vi "Set User Object Tag.vi"(8 "error in (no error)":errorcluster, 9 "Value":variant, 10 "Tag Name":string, 11 "Generic Refnum":refnum<vi>) -> (0 "error out":errorcluster, 1 "Was Tag Set?":bool, 3 "dup Generic Refnum":refnum<vi>)   [LabVIEW 2020, in "UserTags.lvlib"]
doc: "UserTags.lvlib contains VIs that allow you to store data within objects or VIs as \"tags\". You can write, read, and remove tags with these VIs.\n\nSet User Object Tag.vi allows you to specify a tag and its associated data for a VI Server object. The VI returns a value indicating whether or not the tag was set.\n\nNote that you must call Save Instrument on the VI that owns this object in order for the tag to be persisted between VI loads.\n\nAlso note that you cannot store Refnum data or LabVIEW Class data within the value for a tag. Attempting to do so will result in this VI returning Error 1."
uses:
  <vilib>/UserTags/UserTags.lvlib
  <vilib>/Utility/Data Type/NI_Data Type.lvlib
  <vilib>/Utility/Data Type/Type Definitions/Data Type.ctl
panel:
  in  "Invalid Datatype":string="You cannot store Refnum or LabVIEW Class data in a user tag."
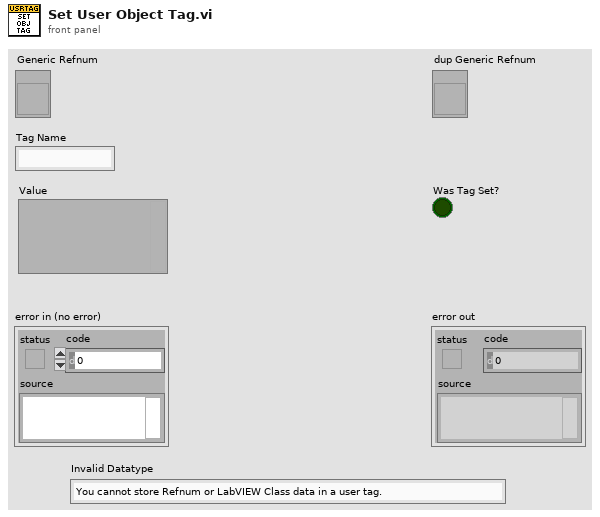
[diagram p1: front panel]
types:
  T1 = typedef "NI_Data Type.lvlib/Data Type.ctl" = enum8{"Invalid Type", "Void", "I8", "I16", "I32", "I64", "U8", "U16", "U32", "U64", "Single Float", "Double Float", "Extended Float", "Single Complex", "Double Complex", "Extended Complex", "Enum U8", "Enum U16", "Enum U32", "Enum U64", "Single Float With Unit", "Double Float With Unit", "Extended Float With Unit", "Single Complex with Unit", "Double Complex with Unit", "Extended Complex with Unit", "Boolean", "String", "Path", "Picture", "Tag", "Array", "Cluster", "Variant", "LV Variant", "Waveform", "Timestamp", "Digital Waveform", "Digital Data", "ExpressData", "Refnum", "External Data", "VI", "Poly VI", "LabVIEW Class Instance", "Fixed Point", "Set Collection", "Map Collection"}
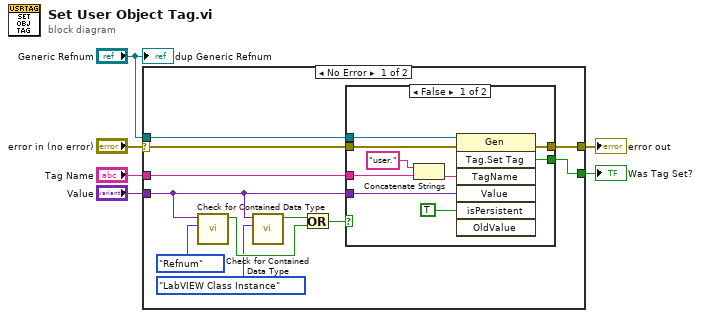
[diagram p0: block diagram]
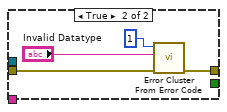
[diagram p2: hidden frame]
diagram:
  n1 = case shown="No Error" "error in (no error)" {
    selector: "error in (no error)" -> [w17 w31]
    tunnel: [w14 w31] -> w5
    tunnel: "Generic Refnum" -> [w16 _]
    tunnel: "Tag Name" -> [w15 _]
    tunnel: [w13 _] -> w2
    tunnel: "Value" -> [w9 _]
    frame No Error {
      n2 = call <vilib>:"Check for Contained Data Type.vi"("data type to find"=Data_Type."Refnum" ("Data Type to Find"), "variant"=w9) -> ("contains data type to find?"=w11:bool)  [unwired: 8 in, 1 out]
      n3 = call <vilib>:"Check for Contained Data Type.vi"("data type to find"=Data_Type."LabVIEW Class Instance" ("Data Type to Find"), "variant"=w9) -> ("contains data type to find?"=w12:bool)  [unwired: 8 in, 1 out]
      n4 = Or(x=w12, y=w11) -> (x .or. y?=w10:bool)
      n5 = case shown="False" w10 {
        tunnel: w17 -> [w26 w27]
        tunnel: w16 -> [w25 _]
        tunnel: w15 -> [w24 _]
        tunnel: [w22 w30] -> w14
        tunnel: [w21 _] -> w13
        tunnel: w9 -> [w20 _]
        frame False {
          n6 = Concatenate Strings("user." ("string"), w24) -> (w18:string)
          n7 = invoke class="Gen" method="Tag.Set Tag"(reference=w25, error in=w26, "TagName"=w18, "Value"=w20, "isPersistent"=TRUE ("Is Persistent?")) -> (error out=w22:errorcluster, "SetTag"=w21:bool)  [unwired: 2 in, 5 out]
        }
        frame True {
          n8 = call <vilib>:"Error Cluster From Error Code.vi"("error in (no error)"=w27, "error message (\"\")"="Invalid Datatype", "error code (0)"=1) -> ("error out"=w30:errorcluster)  [unwired: 6 in]
        }
      }
    }
    frame Error {
    }
  }
  "error out" <- w5
  "Was Tag Set?" <- w2
  "dup Generic Refnum" <- "Generic Refnum"
